vi "MLTH2Odll.vi"(8 "error in (no error)":errorcluster, 9 "p2":dbl, 10 "p1":dbl, 11 "t":dbl) -> (0 "error out":errorcluster, 1 "p2 out":dbl, 2 "p1 out":dbl, 3 "t out":dbl)   [LabVIEW 2016]
doc: "subroutine MLTH2Odll(t, p1, p2)\nCompute melting line of water, see fluid file for reference.\n\nINPUTS:\nt -- Temperature [K]\n\nOUTPUTS:\np1 -- Higher melting line pressure [kPa]\np2-- Lower melting line pressure [kPa] \n\nAbove 273.16 K, only P1 returns a physical answer. Between 251.165 and 273.16 K, two pressures are returned. If flags\nof -998 or -999 are sent for the temperature, the value of the lowest temperature possible (251.165 K) is sent back in t, \nthe pressure at that point is sent back in P1, and the density at that point is sent back in P2 if the flag -998 is used."
uses:
  REFPROP.DLL
panel:
  # "REFPROP-MLTH2Odll.vi"
  # "void  MLTH2Odll(double *t, double *p1, double *p2)"
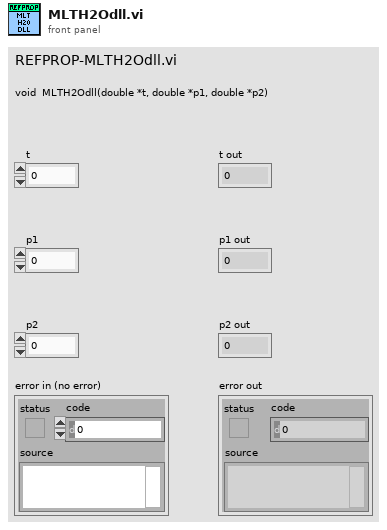
[diagram p1: front panel]
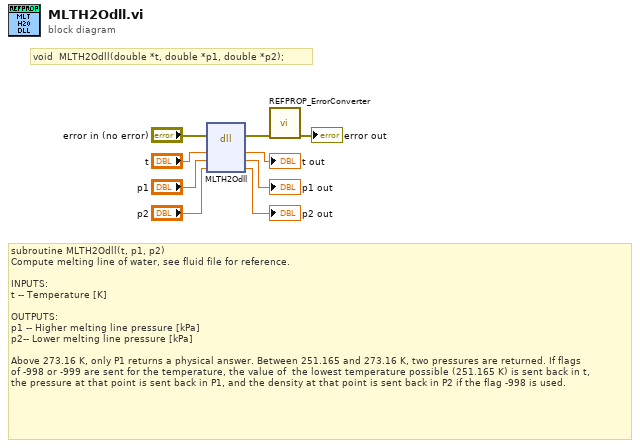
[diagram p0: block diagram]
diagram:
  # "void  MLTH2Odll(double *t, double *p1, double *p2);"
  # "subroutine MLTH2Odll(t, p1, p2)\nCompute melting line of water, see fluid file for reference.\n\nINPUTS:\nt -- Temperature [K]\n\nOUTPUTS:\np1 -- Higher melting line pressure [kPa]\np2-- Lower melting line pressure [kPa] \n\nAbove 273.16 K, only P1 returns a physical answer. Between 251.165 and 273.16 K, two pressures are returned. If flags\nof -998 or -999 are sent for the temperature, the value of  the lowest temperature possible (251.165 K) is sent back in t, \nthe pressure at that point is sent back in P1, and the density at that point is sent back in P2 if the flag -998 is used."
  n1 = dll-call lib="S:/009 - Testing/02 - Performance Testing/REFPROP/REFPROP.*" fn="MLTH2Odll"(error in="error in (no error)", "t"="t", "p1"="p1", "p2"="p2") -> (error out=w3:errorcluster, "t"=→"t out":dbl, "p1"=→"p1 out":dbl, "p2"=→"p2 out":dbl)  [unwired: 3 in, 1 out]
  n2 = call "REFPROP_ErrorConverter.vi"("error in (no error)"=w3) -> ("error out"=→"error out":errorcluster)  [unwired: 10 in]
